vi "UI Main.vi"() -> ()   [LabVIEW 2020]
uses:
  controls/UI Data.ctl
  support/Message Queue/Message Cluster.ctl
  Globals/Global - All UI Loop Stop.vi
  Globals/Global - UI Stream and Variable Connections.vi
  Globals/Global - Configuration Options.vi
  support/User Event - Stop/User Event - Stop.lvlib
  support/Message Queue/Message Queue.lvlib
panel:
  out "Current Logging State":u16(ring) items=["Logging", "Idle (Safe State)"]
  in  "Exit":bool
  out "System Status":string
  in  "Settings Tab":enum32{"UI Commands", "System Monitoring"}(tab)
  in  "Live Data Channel":u32 max=3 step=1
  out "Live Data":waveform(dbl)(graph)
  in  "Stop Live Data":bool
  in  "Acquire Live Data":bool
  out "Most recent manually-triggered log file":path
  in  "Force Trigger":bool
  in  "Unbalanced Fan Speed":fxp<+/-,64,32>
  out "Number of Data Files":u32
  out "Actual Loop Period (ticks)":u32
  out "Largest Contiguous Memory (bytes)":dbl(graph)
  out "Resource Utilization (%)":cluster{dbl, "Double":dbl, dbl}(graph)
  out "System Time":timestamp
  out "Connected?":bool
  in  "Connect to Controller":bool
  in  "Controller Address":string
  # "LabVIEW FPGA Waveform Acquisition and Logging on CompactRIO"
  # "Connection Settings"
  # "Live Data"
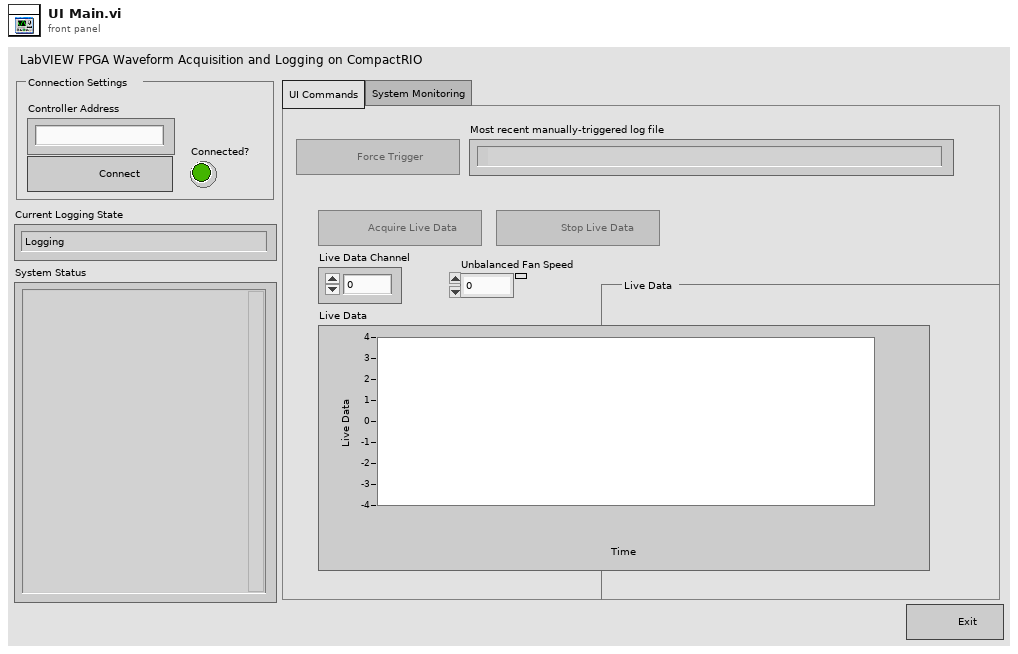
[diagram p1: front panel]
types:
  T1 = typedef "UI Data.ctl" = cluster{"Create Log File Ref":refnum<vi>, "Acquire Live Data Ref":refnum<vi>, "Stop Live Data Ref":refnum<vi>}
  T2 = typedef "Message Queue.lvlib/All Host Message Queues.ctl" = cluster{"UI":refnum<queue>}
  T3 = typedef "Message Queue.lvlib/Message Cluster.ctl" = cluster{"Message":string, "Message Data":variant}
  T4 = typedef "Variable References.ctl" = cluster{"CPU Usage":refnum<k21>, "Contiguous Memory":refnum<k21>, "Actual Loop Period":refnum<k21>, "Buffer Backlog":refnum<k21>, "Drive Space":refnum<k21>, "Number of Data Files":refnum<k21>, "System Time":refnum<k21>}
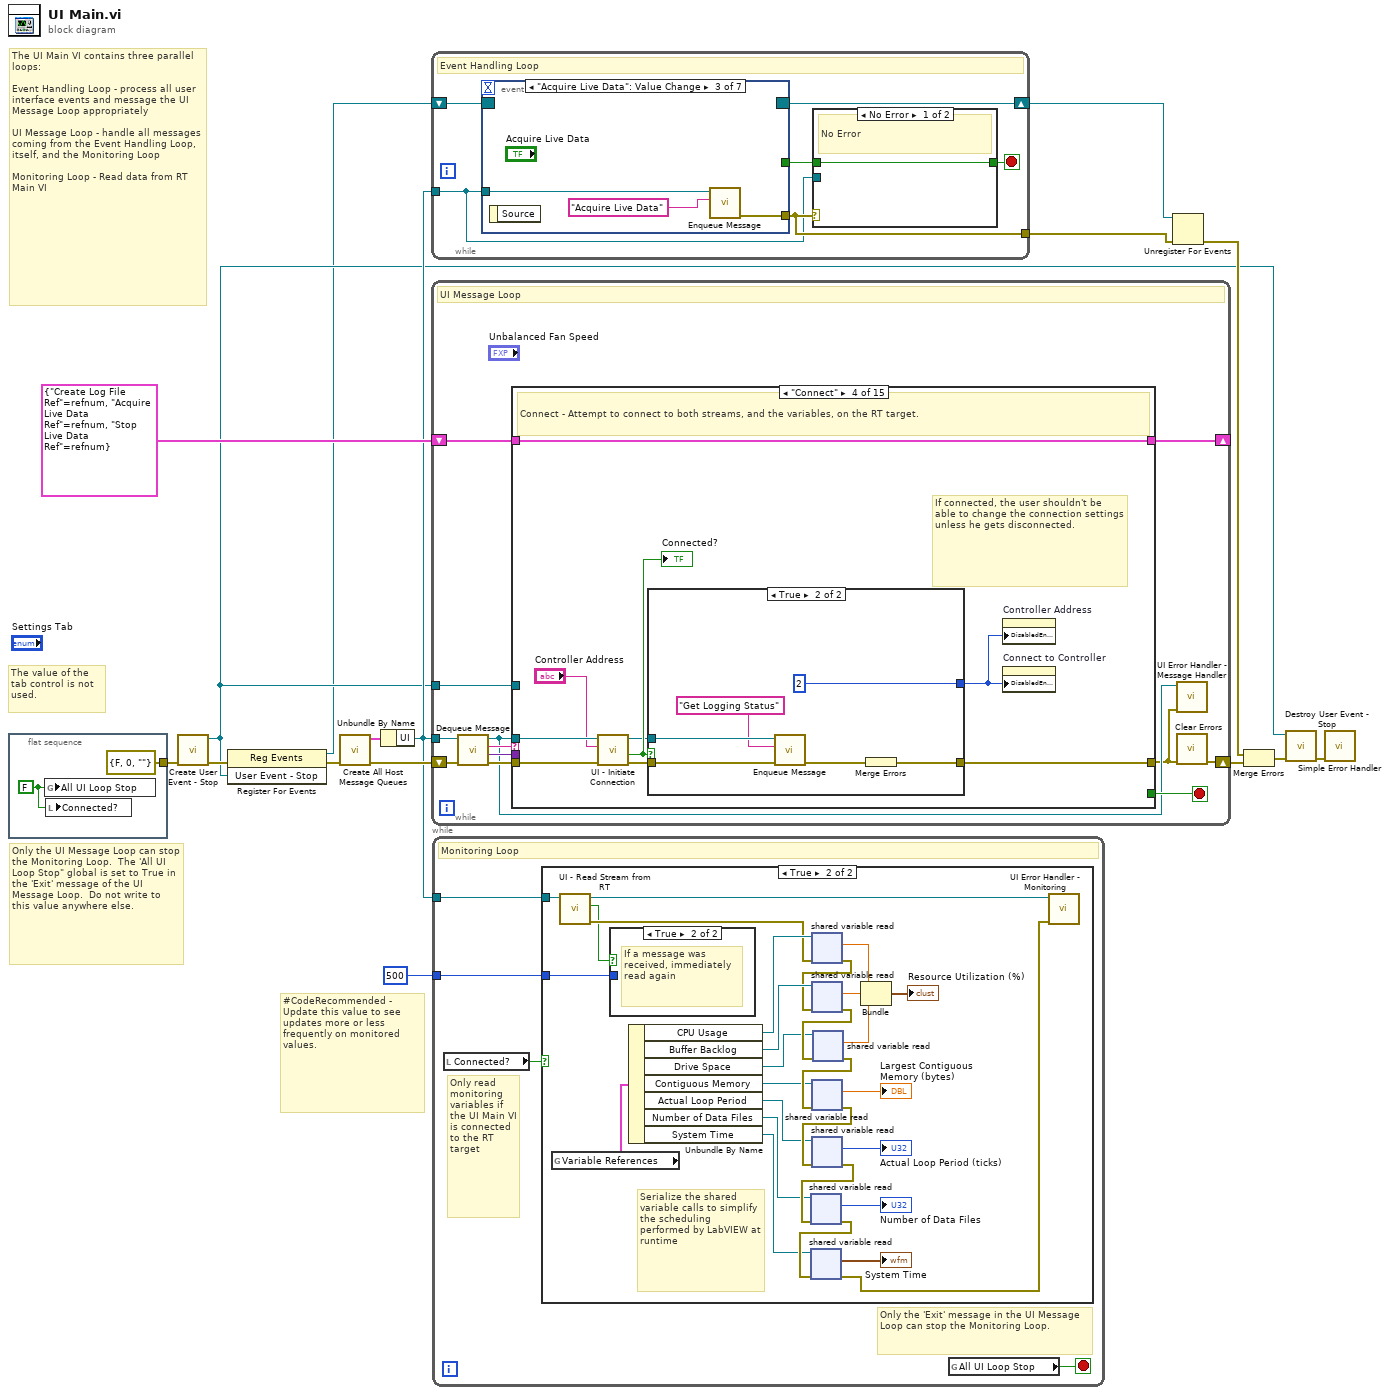
[diagram p0: block diagram]
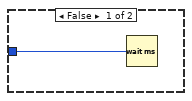
[diagram p2: hidden frame]
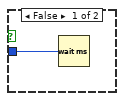
[diagram p3: hidden frame]
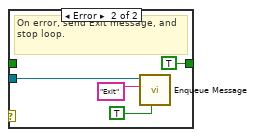
[diagram p4: hidden frame]
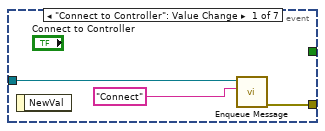
[diagram p5: hidden frame]
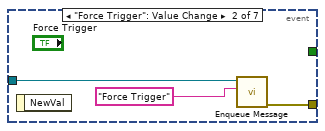
[diagram p6: hidden frame]
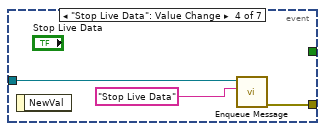
[diagram p7: hidden frame]
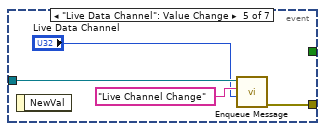
[diagram p8: hidden frame]
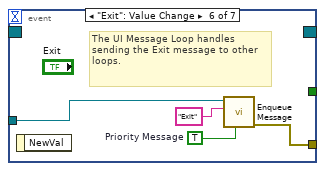
[diagram p9: hidden frame]
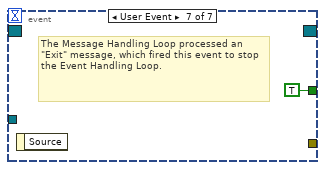
[diagram p10: hidden frame]
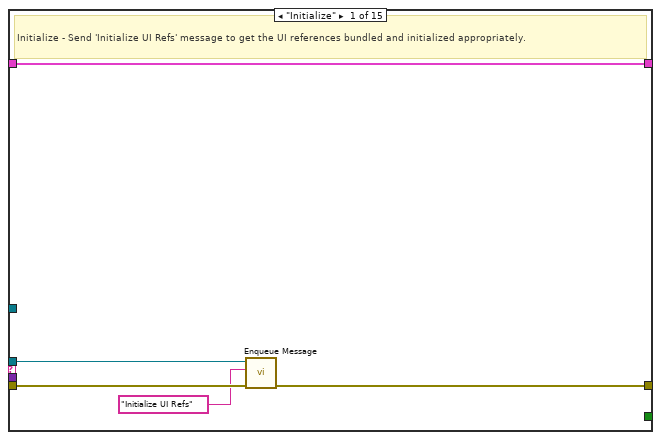
[diagram p11: hidden frame]
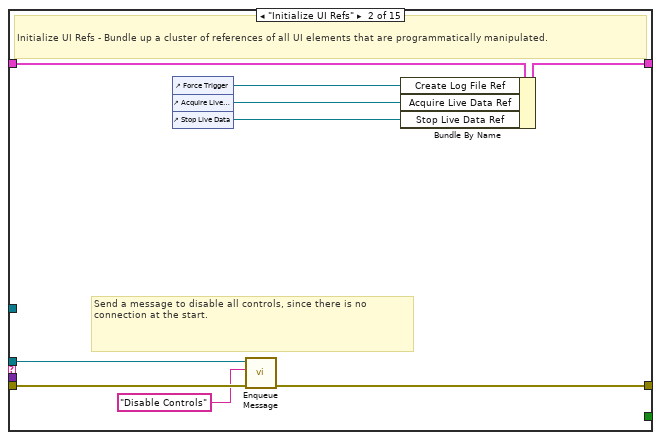
[diagram p12: hidden frame]
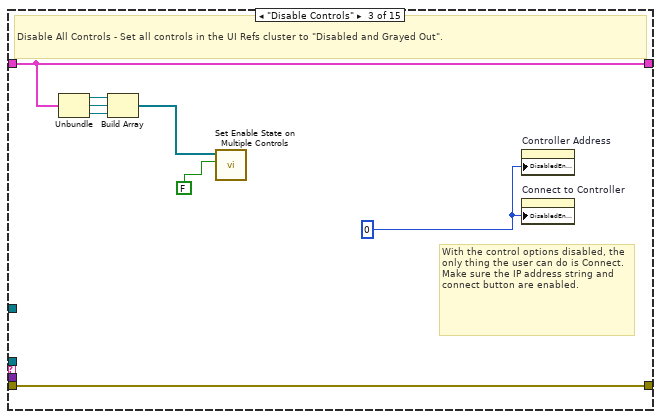
[diagram p13: hidden frame]
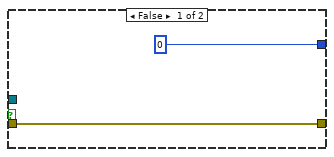
[diagram p14: hidden frame]
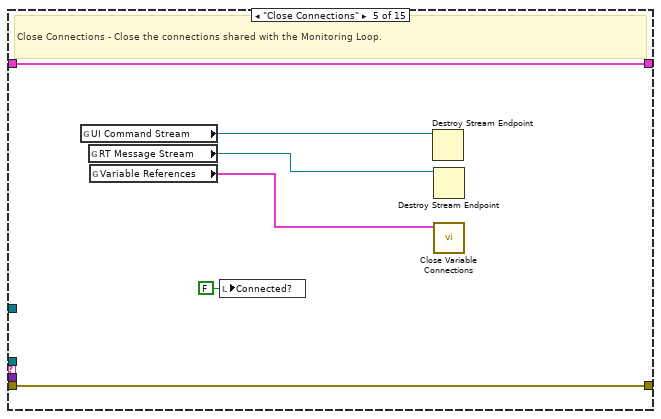
[diagram p15: hidden frame]
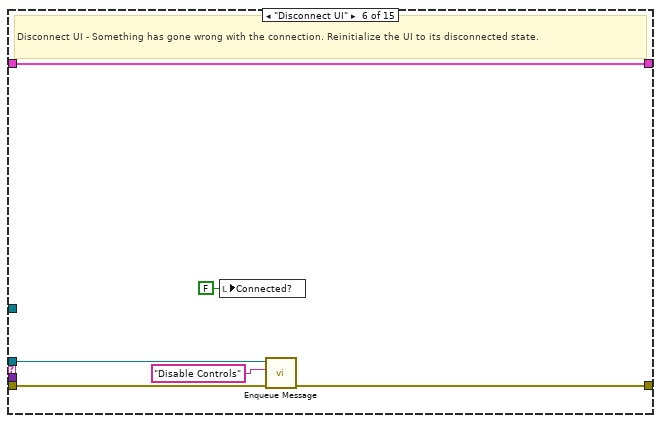
[diagram p16: hidden frame]
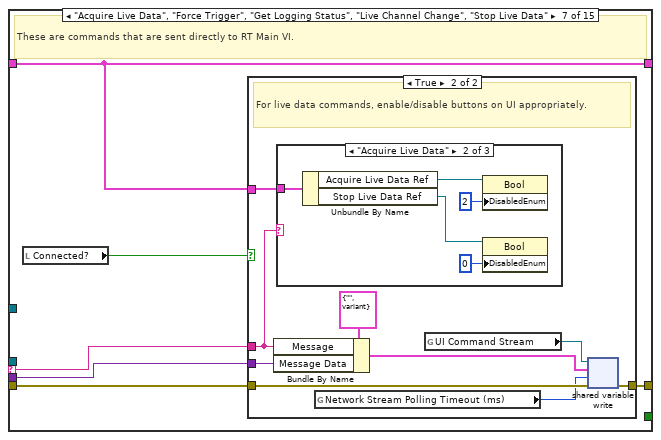
[diagram p17: hidden frame]
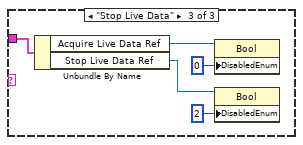
[diagram p20: hidden frame]
diagram:
  # "#CodeRecommended - Update this value to see updates more or less frequently on monitored values."
  # "The UI Main VI contains three parallel loops:\n\nEvent Handling Loop - process all user interface events and message the UI Message Loop appropriately\n\nUI Message Loop - handle all messages coming from the Event Handling Loop, itself, and the Monitoring Loop\n\nMonitoring Loop - Read data from RT Main VI"
  # "The value of the tab control is not used."
  # "Only the UI Message Loop can stop the Monitoring Loop.  The 'All UI Loop Stop\" global is set to True in the 'Exit' message of the UI Message Loop.  Do not write to this value anywhere else."
  n1 = flat-sequence {
    tunnel: [errorcluster {"status"=FALSE, "code"=0, "source"=""} ("error in (no error)")] -> w6
    frame #0 {
      w17 = FALSE
      n2 = global write "Global - All UI Loop Stop.vi" "All UI Loop Stop"(w17) -> ()
      n3 = local write "Connected?"(w17) -> ()
    }
  }
  n4 = call "Create User Event - Stop.vi"("error in (no error)"=w6) -> ("error out"=w4:errorcluster, "User Event - Stop"=w2:refnum<user-event>)  [unwired: 9 in]
  n5 = register-events(error in=w4, w2) -> (reference out=w1:refnum<event-registration>, error out=w3:errorcluster)  [unwired: 1 in]
  n6 = call "Create All Host Message Queues.vi"("error in (no error)"=w3) -> ("error out"=w12:errorcluster, "Message Queues out"=w13:T2)  [unwired: 9 in]
  n7 = Unbundle By Name(w13) -> ("UI"=w7:refnum<queue>)
  n8 = while {
    tunnel: w7 -> [w20]
    tunnel: [w22] -> w15
    shift-right: [w19] -> w10
    shift-left: w1 -> [w21]
    stop <- w23 stop-if-true
    # "Event Handling Loop"
    n9 = event shown="[2] \"Acquire Live Data\": Value Change" {
      selector: w21 -> [_ _ _ _ _ _ _]
      dyn-events: [_ _ _ _ _ _ _] -> w19
      timeout: _ -> [_ _ _ _ _ _ _]
      tunnel: [_ _ _ _ _ _ TRUE ("Discard?")] -> w24
      tunnel: w20 -> [w30 w33 w36 w39 w43 w46 _]
      tunnel: [w32 w35 w38 w41 w45 w49 _] -> w22
      event "Connect to Controller": Value Change {
        n10 = event-data() -> ()  [unwired: 1 in, 1 out]
        n11 = call "Enqueue Message.vi"("Message"="Connect", "Message Queue"=w30) -> ("error out"=w32:errorcluster)  [unwired: 8 in, 1 out]
      }
      event "Force Trigger": Value Change {
        n12 = event-data() -> ()  [unwired: 1 in, 1 out]
        n13 = call "Enqueue Message.vi"("Message"="Force Trigger", "Message Queue"=w33) -> ("error out"=w35:errorcluster)  [unwired: 8 in, 1 out]
      }
      event "Acquire Live Data": Value Change {
        n14 = event-data() -> ()  [unwired: 1 in, 1 out]
        n15 = call "Enqueue Message.vi"("Message"="Acquire Live Data", "Message Queue"=w36) -> ("error out"=w38:errorcluster)  [unwired: 8 in, 1 out]
      }
      event "Stop Live Data": Value Change {
        n16 = event-data() -> ()  [unwired: 1 in, 1 out]
        n17 = call "Enqueue Message.vi"("Message"="Stop Live Data", "Message Queue"=w39) -> ("error out"=w41:errorcluster)  [unwired: 8 in, 1 out]
      }
      event "Live Data Channel": Value Change {
        n18 = event-data() -> ()  [unwired: 1 in, 1 out]
        n19 = call "Enqueue Message.vi"("Message Data"="Live Data Channel", "Message"="Live Channel Change", "Message Queue"=w43) -> ("error out"=w45:errorcluster)  [unwired: 7 in, 1 out]
      }
      event "Exit": Value Change {
        w47 = TRUE  # Priority Message
        # "The UI Message Loop handles sending the Exit message to other loops."
        n20 = event-data() -> ()  [unwired: 1 in, 1 out]
        n21 = call "Enqueue Message.vi"("Priority Message? (F)"=w47, "Message"="Exit", "Message Queue"=w46) -> ("error out"=w49:errorcluster)  [unwired: 7 in, 1 out]
      }
      event User Event {
        # "The Message Handling Loop processed an \"Exit\" message, which fired this event to stop the Event Handling Loop."
        n22 = event-data() -> ()  [unwired: 1 in, 1 out]
      }
    }
    n23 = case shown="No Error" w22 {
      tunnel: [w25 TRUE ("Discard?")] -> w23
      tunnel: w24 -> [w25 _]
      tunnel: w20 -> [_ w26]
      frame No Error {
        # "No Error"
      }
      frame Error {
        # "On error, send Exit message, and stop loop."
        n24 = call "Enqueue Message.vi"("Priority Message? (F)"=TRUE ("Discard?"), "Message"="Exit", "Message Queue"=w26) -> ()  [unwired: 7 in, 2 out]
      }
    }
  }
  n25 = while {
    tunnel: w7 -> [w56]
    tunnel: w2 -> [w61]
    shift-right: [w51] -> w16
    shift-left: w12 -> [w60]
    shift-right: [w54] -> _
    shift-left: T1 {"Create Log File Ref"=refnum, "Acquire Live Data Ref"=refnum, "Stop Live Data Ref"=refnum} ("Measurement UI Controls") -> [w55]
    stop <- w62 stop-if-true
    # "UI Message Loop"
    n26 = call "Dequeue Message.vi"("error in (no error)"=w60, "Message Queue"=w56) -> ("error out"=w59:errorcluster, "Message Data"=w57:variant, "Message"=w58:string, "dup Message Queue"=w53:refnum<queue>)  [unwired: 6 in]
    n27 = case "Message Cases" shown="\"Connect\"" w58 {
      selector: w58 -> [_ _ _ _ _ _ w116 _ _ _ w168 _ _ _ w229]
      tunnel: w53 -> [w64 w72 _ w92 _ w109 _ _ _ _ w172 _ w214 _ _]
      tunnel: w59 -> [w66 w76 w84 w93 w107 w111 w119 w145 w151 w166 w182 w203 w219 w224 _]
      tunnel: [w65 w73 w84 w87 w107 w110 w118 w143 w149 w165 w183 w201 w220 w223 w227] -> w52
      tunnel: [_ _ _ _ _ _ _ _ _ _ _ _ TRUE _ _] -> w62
      tunnel: w57 -> [_ _ _ _ _ _ w117 w142 w148 w164 w180 w200 _ _ _]
      tunnel: w61 -> [_ _ _ _ _ _ _ _ _ _ _ _ w218 _ _]
      tunnel: w55 -> [w67 w75 w83 w91 w106 w113 w115 w144 w150 w159 w184 w202 w216 w222 w225]
      tunnel: [w67 w74 w83 w91 w106 w113 w115 w144 w150 w159 w184 w202 w216 w222 w225] -> w54
      frame "Initialize" {
        # "Initialize - Send 'Initialize UI Refs' message to get the UI references bundled and initialized appropriately."
        n28 = call "Enqueue Message.vi"("error in (no error)"=w66, "Message"="Initialize UI Refs", "Message Queue"=w64) -> ("error out"=w65:errorcluster)  [unwired: 7 in, 1 out]
      }
      frame "Initialize UI Refs" {
        # "Send a message to disable all controls, since there is no connection at the start."
        # "Initialize UI Refs - Bundle up a cluster of references of all UI elements that are programmatically manipulated."
        n29 = control-ref of="Force Trigger"() -> (w70:refnum<vi>)
        n30 = control-ref of="Acquire Live Data"() -> (w69:refnum<vi>)
        n31 = control-ref of="Stop Live Data"() -> (w68:refnum<vi>)
        n32 = call "Enqueue Message.vi"("error in (no error)"=w76, "Message"="Disable Controls", "Message Queue"=w72) -> ("error out"=w73:errorcluster)  [unwired: 7 in, 1 out]
        n33 = Bundle By Name(cluster=w75, "Create Log File Ref"=w70, "Acquire Live Data Ref"=w69, "Stop Live Data Ref"=w68) -> (w74:T1)
      }
      frame "Disable Controls" {
        w79 = 0
        # "With the control options disabled, the only thing the user can do is Connect. Make sure the IP address string and connect button are enabled."
        # "Disable All Controls - Set all controls in the UI Refs cluster to \"Disabled and Grayed Out\"."
        n34 = Unbundle(w83) -> ("Create Log File Ref"=w82:refnum<vi>, "Acquire Live Data Ref"=w78:refnum<vi>, "Stop Live Data Ref"=w77:refnum<vi>)
        n35 = Build Array(w82, w78, w77) -> (w81:refnum<vi>[])
        n36 = call "Set Enable State on Multiple Controls.vi"("Enable?"=FALSE, "Controls"=w81) -> ()  [unwired: 10 in]
        n37 = property on="Controller Address" class="Str"("DisabledEnum"=w79) -> ()  [unwired: 2 in, 2 out]
        n38 = property on="Connect to Controller" class="Bool"("DisabledEnum"=w79) -> ()  [unwired: 2 in, 2 out]
      }
      frame "Connect" {
        # "If connected, the user shouldn't be able to change the connection settings unless he gets disconnected."
        # "Connect - Attempt to connect to both streams, and the variables, on the RT target."
        n39 = call "UI - Initiate Connection.vi"("error in (no error)"=w93, "Controller Address"="Controller Address", "Message Queue"=w92) -> ("error out"=w89:errorcluster, "Connected?"=w88:bool, "dup Message Queue"=w86:refnum<queue>)  [unwired: 6 in]
        "Connected?" <- w88
        n40 = case shown="True" w88 {
          tunnel: w89 -> [w95 w100]
          tunnel: [w95 w96] -> w87
          tunnel: w86 -> [_ w99]
          tunnel: [0 2] -> w85
          frame False {
          }
          frame True {
            n41 = call "Enqueue Message.vi"("error in (no error)"=w100, "Message"="Get Logging Status", "Message Queue"=w99) -> ("error out"=w101:errorcluster)  [unwired: 7 in, 1 out]
            n42 = Merge Errors(w101) -> (w96:errorcluster)
          }
        }
        n43 = property on="Controller Address" class="Str"("DisabledEnum"=w85) -> ()  [unwired: 2 in, 2 out]
        n44 = property on="Connect to Controller" class="Bool"("DisabledEnum"=w85) -> ()  [unwired: 2 in, 2 out]
      }
      frame "Close Connections" {
        # "Close Connections - Close the connections shared with the Monitoring Loop."
        n45 = global read "Global - UI Stream and Variable Connections.vi" "UI Command Stream"() -> (w105:refnum<k21>)
        n46 = global read "Global - UI Stream and Variable Connections.vi" "RT Message Stream"() -> (w104:refnum<k21>)
        n47 = global read "Global - UI Stream and Variable Connections.vi" "Variable References"() -> (w103:T4)
        n48 = local write "Connected?"(FALSE ("Connected?")) -> ()
        n49 = Destroy Stream Endpoint(11:w105) -> ()  [unwired: 1 in, 1 out]
        n50 = Destroy Stream Endpoint(11:w104) -> ()  [unwired: 1 in, 1 out]
        n51 = call "Close Variable Connections.vi"("Variable References"=w103) -> ()  [unwired: 11 in]
      }
      frame "Disconnect UI" {
        # "Disconnect UI - Something has gone wrong with the connection. Reinitialize the UI to its disconnected state."
        n52 = local write "Connected?"(FALSE ("Connected?")) -> ()
        n53 = call "Enqueue Message.vi"("error in (no error)"=w111, "Message"="Disable Controls", "Message Queue"=w109) -> ("error out"=w110:errorcluster)  [unwired: 7 in, 1 out]
      }
      frame "Acquire Live Data", "Force Trigger", "Get Logging Status", "Live Channel Change", "Stop Live Data" {
        # "These are commands that are sent directly to RT Main VI."
        n54 = local read "Connected?"() -> (w114:bool)
        n55 = case shown="True" w114 {
          tunnel: w119 -> [w120 w129]
          tunnel: [w120 w128] -> w118
          tunnel: w117 -> [_ w123]
          tunnel: w116 -> [_ w121]
          tunnel: w115 -> [_ w122]
          frame False {
            # "Don't bother trying to send a message to the RT system if UI Main VI isn't even connected"
          }
          frame True {
            # "For live data commands, enable/disable buttons on UI appropriately."
            n56 = Bundle By Name(cluster=T3 {"Message"="", "Message Data"=variant} ("Message Cluster"), "Message"=w121, "Message Data"=w123) -> (w124:T3)
            n57 = case shown="\"Acquire Live Data\"" w121 {
              tunnel: w122 -> [_ w134 w139]
              frame Default {
              }
              frame "Acquire Live Data" {
                n58 = Unbundle By Name(w134) -> ("Acquire Live Data Ref"=w133:refnum<vi>, "Stop Live Data Ref"=w132:refnum<vi>)
                n59 = property class="Bool"(reference=w133, "DisabledEnum"=u8 2) -> ()  [unwired: 1 in, 2 out]
                n60 = property class="Bool"(reference=w132, "DisabledEnum"=u8 0) -> ()  [unwired: 1 in, 2 out]
              }
              frame "Stop Live Data" {
                n61 = Unbundle By Name(w139) -> ("Acquire Live Data Ref"=w138:refnum<vi>, "Stop Live Data Ref"=w137:refnum<vi>)
                n62 = property class="Bool"(reference=w138, "DisabledEnum"=u8 0) -> ()  [unwired: 1 in, 2 out]
                n63 = property class="Bool"(reference=w137, "DisabledEnum"=u8 2) -> ()  [unwired: 1 in, 2 out]
              }
            }
            n64 = global read "Global - Configuration Options.vi" "Network Stream Polling Timeout (ms)"() -> (w126:i32)
            n65 = global read "Global - UI Stream and Variable Connections.vi" "UI Command Stream"() -> (w127:refnum<k21>)
            n66 = shared-variable-write(w127, w129, w124, w126) -> (w128:errorcluster)  [unwired: 2 out]
          }
        }
      }
      frame "Send Path to UI" {
        # "Send Path to UI - Message from the RT Main VI containing the path to the manually-triggered log file."
        n67 = Variant To Data(error in=w145, type=path "", Variant=w142) -> (data=→"Most recent manually-triggered log file":path, error out=w143:errorcluster)
      }
      frame "Send Live Data to UI" {
        # "Send Live Data to UI - Message from the RT Main VI containing the latest live data for the specified channel."
        n68 = Variant To Data(error in=w151, type=waveform(dbl) {"t0"=timestamp(0 s since 1904-01-01), "dt"=1.0, "Y"=[]}, Variant=w148) -> (data=→"Live Data":waveform(dbl), error out=w149:errorcluster)
      }
      frame "Send Logging Status" {
        # "TRUE: Logging Normally\nFALSE: Idle (Safe State)"
        # "Send Logging Status - Message from the RT Main VI indicating whether or not logging is happening normally, or if the logging loop is in safe mode."
        n69 = Unbundle By Name(w159) -> ("Create Log File Ref"=w158:refnum<vi>, "Acquire Live Data Ref"=w157:refnum<vi>, "Stop Live Data Ref"=w153:refnum<vi>)
        n70 = Variant To Data(error in=w166, type=FALSE, Variant=w164) -> (data=w154:bool, error out=w165:errorcluster)
        n71 = Build Array(w158, w157) -> (w156:refnum<vi>[])
        n72 = Build Array(w153) -> (w155:refnum<vi>[])
        n73 = Select(t=u16 0, s=w154, f=u16 1) -> (s? t:f=→"Current Logging State":u16)
        n74 = call "Set Enable State on Multiple Controls.vi"("Enable?"=w154, "Controls"=w156) -> ()  [unwired: 10 in]
        n75 = call "Set Enable State on Multiple Controls.vi"("Enable?"=FALSE, "Controls"=w155) -> ()  [unwired: 10 in]
      }
      frame "Critical Error", "Log-Only Error", "Non-Critical Error", "RT Error" {
        # "Error - Display message in status indicator on panel.  If it's a critical error, shut down this VI with an 'Exit' message."
        n76 = case shown="Default" w168 {
          selector: w168 -> [_ w186]
          tunnel: ["UI Error" w186] -> w167
          frame Default {
          }
          frame "RT Error" {
          }
        }
        n77 = Variant To Data(error in=w182, type=errorcluster {"status"=FALSE, "code"=0, "source"=""} ("error constant"), Variant=w180) -> (data=w175:errorcluster, error out=w181:errorcluster)
        n78 = Unbundle By Name(w175) -> ("code"=w174:i32, "source"=w178:string)
        n79 = Format Date/Time String() -> (date/time string=w177:string)  [unwired: 3 in]
        n80 = Format Into String(format string="\n%s: %s %d - %s", w177, w167, w174, w178) -> (resulting string=w169:string)  [unwired: 2 in, 1 out]
        n81 = call "Enqueue Message.vi"("error in (no error)"=w181, "Message Data"=w169, "Message"="Update System Status", "Message Queue"=w172) -> ("error out"=w173:errorcluster, "dup Message Queue"=w171:refnum<queue>)  [unwired: 6 in]
        n82 = case shown="Default" w168 {
          tunnel: w173 -> [w187 w191]
          tunnel: w171 -> [_ w189]
          tunnel: [w187 w190] -> w183
          frame Default {
          }
          frame "Critical Error" {
            n83 = call "Enqueue Message.vi"("error in (no error)"=w191, "Message"="Exit", "Message Queue"=w189) -> ("error out"=w190:errorcluster)  [unwired: 7 in, 1 out]
          }
        }
      }
      frame "Update System Status" {
        # "#CodeRecommended - The code below ensures that the System Status string value does not become too large.  It uses the same maximum size as the RT error log to determine whether or not to remove the last half of the log string. Change this logic if you wish to maintain more/less of the information in the System Status string."
        # "Update System Status - Add a new string to the beginning of the System Status string on the UI."
        n84 = Variant To Data(error in=w203, type="", Variant=w200) -> (data=w197:string, error out=w201:errorcluster)
        n85 = global read "Global - Configuration Options.vi" "Error Log Max Size (bytes)"() -> (w193:i64)
        n86 = local read "System Status"() -> (w195:string)
        n87 = String Length(string=w195) -> (length=w196:i32)
        n88 = Greater?(x=w196, y=w193) -> (0:w194:bool)
        n89 = case shown="True" w194 {
          tunnel: w195 -> [w204 w208]
          tunnel: w193 -> [_ w207]
          tunnel: [w204 w209] -> w192
          frame False {
          }
          frame True {
            n90 = Divide(x=w207, y=i64 2) -> (x/y=w206:dbl)
            n91 = String Subset(string=w208, length (rest)=w206) -> (substring=w209:string)  [unwired: 1 in]
          }
        }
        n92 = Concatenate Strings(w197, w192) -> (→"System Status":string)
      }
      frame "Exit" {
        # "Close all connections"
        # "Stop Monitoring Loop"
        # "Stop Event Handling Loop"
        # "Release the UI Message queue reference"
        # "Stop UI Message Loop"
        # "Exit - Fire the User Event to stop the Event Handling Loop, and toggle the local variable to stop the Monitoring Loop.  This message alone causes all three loops to stop."
        n93 = global write "Global - All UI Loop Stop.vi" "All UI Loop Stop"(TRUE ("Stop Monitoring Loop")) -> ()
        n94 = call "Fire User Event - Stop.vi"("User Event - Stop"=w218) -> ("error out"=w217:errorcluster)  [unwired: 10 in]
        n95 = Release Queue(queue=w214, error in (no error)=w219) -> (error out=w215:errorcluster)  [unwired: 1 in, 2 out]
        n96 = global read "Global - UI Stream and Variable Connections.vi" "UI Command Stream"() -> (w212:refnum<k21>)
        n97 = global read "Global - UI Stream and Variable Connections.vi" "RT Message Stream"() -> (w211:refnum<k21>)
        n98 = global read "Global - UI Stream and Variable Connections.vi" "Variable References"() -> (w210:T4)
        n99 = Destroy Stream Endpoint(11:w212) -> ()  [unwired: 1 in, 1 out]
        n100 = Destroy Stream Endpoint(11:w211) -> ()  [unwired: 1 in, 1 out]
        n101 = call "Close Variable Connections.vi"("Variable References"=w210) -> ()  [unwired: 11 in]
        n102 = Merge Errors(w217, w215) -> (w220:errorcluster)
      }
      frame "---Copy This Frame---" {
        # "Duplicate this frame when creating new messages.  Change this comment in the duplicated frame to describe this message."
        n103 = Merge Errors(w224) -> (w223:errorcluster)
      }
      frame Default {
        # "'Default' case only runs if there is a message that isn't defined in any of the other cases.  Output a programming error."
        n104 = Format Into String(format string="The invalid message string \"%s\" was received in the Message Handling Loop." ("Invalid Message Loop Message"), w229) -> (resulting string=w226:string)  [unwired: 2 in, 1 out]
        n105 = call <vilib>:"Error Cluster From Error Code.vi"("error message (\"\")"=w226, "error code (0)"=1) -> ("error out"=w227:errorcluster)  [unwired: 7 in]
      }
    }
    n106 = call "UI Error Handler - Message Handler.vi"("error in (no error)"=w52, "Message Queue"=w53) -> ()  [unwired: 9 in, 1 out]
    n107 = call <vilib>:"Clear Errors.vi"("error in (no error)"=w52) -> ("error out"=w51:errorcluster)  [unwired: 5 in, 1 out]
  }
  n108 = while {
    tunnel: w7 -> [w233]
    tunnel: u32 500 ("milliseconds to wait") -> [w231]
    stop <- w234 stop-if-true
    # "Only read monitoring variables if the UI Main VI is connected to the RT target"
    # "Only the 'Exit' message in the UI Message Loop can stop the Monitoring Loop."
    # "Monitoring Loop"
    n109 = local read "Connected?"() -> (w232:bool)
    n110 = case shown="True" w232 {
      tunnel: w233 -> [_ w259]
      tunnel: w231 -> [w235 w236]
      frame False {
        n111 = Wait (ms)(milliseconds to wait=w235) -> ()  [unwired: 1 out]
      }
      frame True {
        # "Serialize the shared variable calls to simplify the scheduling performed by LabVIEW at runtime"
        n112 = global read "Global - UI Stream and Variable Connections.vi" "Variable References"() -> (w257:T4)
        n113 = call "UI - Read Stream from RT.vi"("Message Queue"=w259) -> ("error out"=w260:errorcluster, "Message Received?"=w237:bool, "dup Message Queue"=w258:refnum<queue>)  [unwired: 8 in]
        n114 = case shown="True" w237 {
          tunnel: w236 -> [w264 _]
          frame False {
            n115 = Wait (ms)(milliseconds to wait=w264) -> ()  [unwired: 1 out]
          }
          frame True {
            # "If a message was received, immediately read again"
          }
        }
        n116 = Unbundle By Name(w257) -> ("CPU Usage"=w262:refnum<k21>, "Buffer Backlog"=w261:refnum<k21>, "Drive Space"=w238:refnum<k21>, "Contiguous Memory"=w249:refnum<k21>, "Actual Loop Period"=w246:refnum<k21>, "Number of Data Files"=w243:refnum<k21>, "System Time"=w239:refnum<k21>)
        n117 = shared-variable-read(w262, w260) -> (w256:errorcluster, w254:dbl)  [unwired: 2 out]
        n118 = shared-variable-read(w261, w256) -> (w255:errorcluster, w253:dbl)  [unwired: 2 out]
        n119 = shared-variable-read(w238, w255) -> (w250:errorcluster, w252:dbl)  [unwired: 2 out]
        n120 = shared-variable-read(w249, w250) -> (w247:errorcluster, →"Largest Contiguous Memory (bytes)":dbl)  [unwired: 2 out]
        n121 = shared-variable-read(w246, w247) -> (w245:errorcluster, →"Actual Loop Period (ticks)":u32)  [unwired: 2 out]
        n122 = shared-variable-read(w243, w245) -> (w242:errorcluster, →"Number of Data Files":u32)  [unwired: 2 out]
        n123 = shared-variable-read(w239, w242) -> (w240:errorcluster, →"System Time":timestamp)  [unwired: 2 out]
        n124 = Bundle(w254, "Double"=w253, w252) -> (→"Resource Utilization (%)":cluster{dbl, "Double":dbl, dbl})  [unwired: 1 in]
        n125 = call "UI Error Handler - Monitoring.vi"("error in (no error)"=w240, "Message Queue"=w258) -> ()  [unwired: 9 in, 1 out]
      }
    }
    n126 = global read "Global - All UI Loop Stop.vi" "All UI Loop Stop"() -> (w234:bool)
  }
  n127 = Unregister For Events(event registration refnum=w10, error in=w15) -> (error out=w11:errorcluster)
  n128 = Merge Errors(w11, w16) -> (w14:errorcluster)
  n129 = call "Destroy User Event - Stop.vi"("error in (no error)"=w14, "User Event - Stop"=w2) -> ("error out"=w8:errorcluster)  [unwired: 9 in]
  n130 = call <vilib>:"Simple Error Handler.vi"("error in (no error)"=w8) -> ()  [unwired: 4 in, 5 out]
